vi "Get_ValidGFGVar_List.vi"(8 "Error In":errorcluster) -> (0 "Error Out":errorcluster, 3 "All Variable Names Out":string[](array[string]))   [LabVIEW 2012]
doc: "SciScan 1.2 160622\nThis VI gets the list of GFG Variables that are permitted to be modified by the user\n(For use with the Generic command in the Maccro Module)"
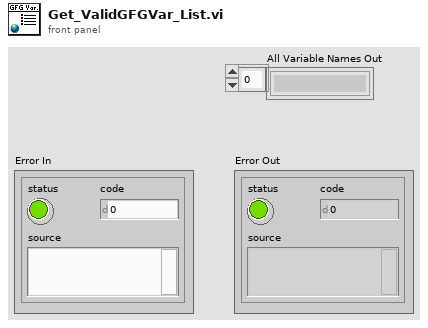
[diagram p1: front panel]
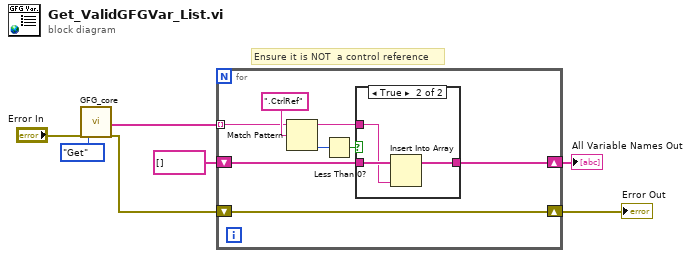
[diagram p0: block diagram]
diagram:
  # "Ensure it is NOT  a control reference"
  n1 = call "GFG_core.vi"("error in (no error)"="Error In", "Action"=enum16{"Init", "Set", "Get", "Clear"}."Get") -> ("All Variable Names Out"=w5:string[], "error out"=w3:errorcluster)  [unwired: 11 in, 5 out]
  n2 = for {
    tunnel: w5 -> [w10] mode=indexing
    shift-right: [w9] -> w1
    shift-left: string[] [] ("All Variable Names Out") -> [w11]
    shift-right: [w8] -> w2
    shift-left: w3 -> [w8]
    n3 = Match Pattern(string=w10, regular expression=".CtrlRef") -> (offset past match=w13:i32)  [unwired: 1 in, 3 out]
    n4 = Less Than 0?(x=w13) -> (x < 0?=w12:bool)
    n5 = case shown="True" w12 {
      tunnel: w11 -> [w15 w18]
      tunnel: w10 -> [_ w17]
      tunnel: [w15 w16] -> w9
      frame False {
      }
      frame True {
        n6 = Insert Into Array(array=w18, new element=w17) -> (w16:string[])  [unwired: 1 in]
      }
    }
  }
  "Error Out" <- w2
  "All Variable Names Out" <- w1
